vi "ARGBSetChannelCore.vi"(7 "Channels":T1, 8 "error in (no error)":errorcluster, 10 "Channel Data in":T2, 11 "Image in":T3) -> (0 "error out":errorcluster)   [LabVIEW 2020, in "image.lvlib"]
uses:
  image.lvlib
  ARGB Image.ctl
  Greyscale Image.ctl
  ARGBChannels.ctl
  common/common.lvlib
  common/bin/gartoolkit_32-1.dll
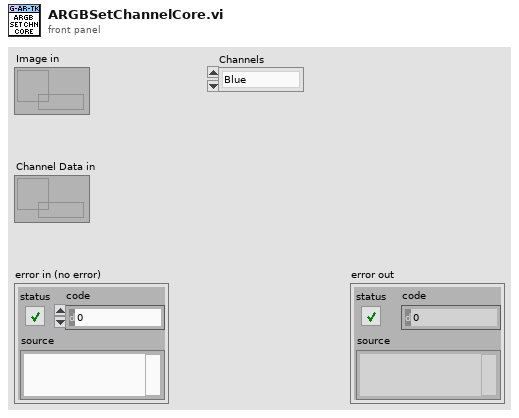
[diagram p1: front panel]
types:
  T1 = typedef "image.lvlib/ARGBChannels.ctl" = enum8{"Blue", "Green", "Red", "Alpha"}
  T2 = typedef "image.lvlib/Greyscale Image.ctl" = refnum<data-value>
  T3 = typedef "image.lvlib/ARGB Image.ctl" = refnum<data-value>
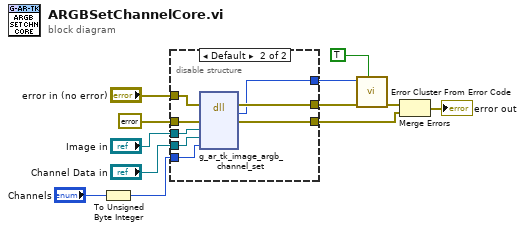
[diagram p0: block diagram]
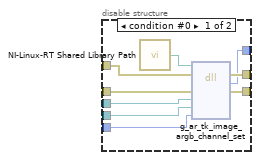
[diagram p2: hidden frame]
diagram:
  n1 = To Unsigned Byte Integer(number="Channels") -> (unsigned 8bit integer=w5:u8)
  n2 = disable-structure shown="Default" {
    disable-tunnel: "error in (no error)" -> [w21 w29]
    disable-tunnel: errorcluster {"status"=FALSE, "code"=0, "source"=""} ("error constant") -> [w20 w28]
    disable-tunnel: "Image in" -> [w19 w27]
    disable-tunnel: "Channel Data in" -> [w18 w26]
    disable-tunnel: w5 -> [w17 w25]
    disable-tunnel: [w16 w24] -> w4
    disable-tunnel: [w15 w23] -> w3
    disable-tunnel: [w14 w22] -> w2
    frame condition #0 {
      n3 = call "NI-Linux-RT Shared Library Path.vi"() -> ("Path"=w13:path)
      n4 = dll-call lib="?" fn="g_ar_tk_image_argb_channel_set" ("g_ar_toolkit.*.*:g_ar_tk_image_draw_picture")(path in=w13, error in=w21, "error_cluster"=w20, "EDVR src"=w19, "EDVR channel data"=w18, "Channel"=w17) -> (error out=w16:errorcluster, "MgErr"=w15:i32, "error_cluster"=w14:errorcluster)  [unwired: 4 in, 1 out]
    }
    frame condition #1 (active) {
      n5 = dll-call lib="C:/serenial/lib/g-augmented-reality-toolkit/LabVIEW/common/bin/gartoolkit_*-1.*" fn="g_ar_tk_image_argb_channel_set" ("g_ar_toolkit.*.*:g_ar_tk_image_draw_picture")(error in=w29, "error_cluster"=w28, "EDVR src"=w27, "EDVR channel data"=w26, "Channel"=w25) -> (error out=w24:errorcluster, "MgErr"=w23:i32, "error_cluster"=w22:errorcluster)  [unwired: 5 in, 1 out]
    }
  }
  n6 = call <vilib>:"Error Cluster From Error Code.vi"("show call chain? (False)"=TRUE, "error in (no error)"=w4, "error code (0)"=w3) -> ("error out"=w11:errorcluster)  [unwired: 6 in]
  n7 = Merge Errors(w11, w2) -> (→"error out":errorcluster)
